vi "Find First Error.vi"(0 "error in (no error)":errorcluster, 1 "source messages":string, 3 "error codes":i32[](array[numeric])) -> (2 "error out":errorcluster, 5 "error?":bool)   [LabVIEW 2014]
doc: "Tests the error status of one or more low-level functions or subVIs that produce a numeric error code as output."
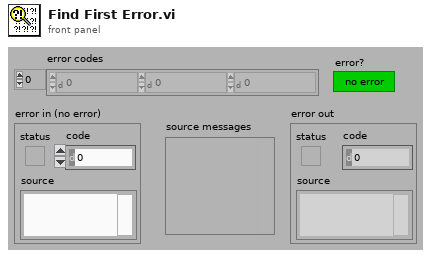
[diagram p1: front panel]
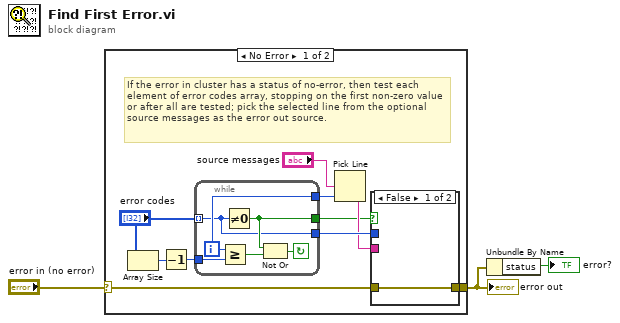
[diagram p0: block diagram]
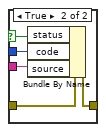
[diagram p2: hidden frame]
diagram:
  n1 = case shown="No Error" "error in (no error)" {
    selector: "error in (no error)" -> [w4 w26]
    tunnel: [w8 w26] -> w1
    frame No Error {
      # "If the error in cluster has a status of no-error, then test each element of error codes array, stopping on the first non-zero value or after all are tested; pick the selected line from the optional source messages as the error out source."
      n2 = Array Size(array="error codes") -> (size(s)=w9:i32)
      n3 = Decrement(x=w9) -> (x-1=w10:i32)
      n4 = while {
        tunnel: w10 -> [w15]
        tunnel: "error codes" -> [w14] mode=indexing
        tunnel: [w16] -> w13
        tunnel: [w17] -> w5
        tunnel: [w14] -> w7
        i -> [w16]
        stop <- w18 continue-if-true
        n5 = Greater Or Equal?(x=w16, y=w15) -> (x >= y?=w19:bool)
        n6 = Not Equal To 0?(x=w14) -> (x != 0?=w17:bool)
        n7 = Not Or(1:w19, 2:w17) -> (0:w18:bool)
      }
      n8 = Pick Line(multi-line string="source messages", line index=w13) -> (output string=w6:string)  [unwired: 1 in]
      n9 = case shown="False" w5 {
        selector: w5 -> [_ w23]
        tunnel: w4 -> [w20 w25]
        tunnel: [w20 w24] -> w8
        tunnel: w7 -> [_ w22]
        tunnel: w6 -> [_ w21]
        frame False {
        }
        frame True {
          n10 = Bundle By Name(cluster=w25, "status"=w23, "code"=w22, "source"=w21) -> (w24:errorcluster)
        }
      }
    }
    frame Error {
      # "If the error in cluster has a status of ERROR, pass it through without test for local errors"
    }
  }
  "error out" <- w1
  n11 = Unbundle By Name(w1) -> ("status"=→"error?":bool)
